vi "Port_set.vi"(8 "error in (no error)":errorcluster, 9 "Port":i32=10002 min=1, 10 "Stream Group":i32=1 min=1, 11 "OXY_SCPI Reseource In":refnum<visa-resource-name>) -> (0 "error out":errorcluster, 1 "communication_data":T1, 3 "OXY_SCPI Reseource Out":refnum<visa-resource-name>)   [LabVIEW 2020, in "OXYGEN_Datastream.lvlib"]
uses:
  OXYGEN_Datastream.lvlib
  TypeDefs/Cluster_RawCommData.ctl
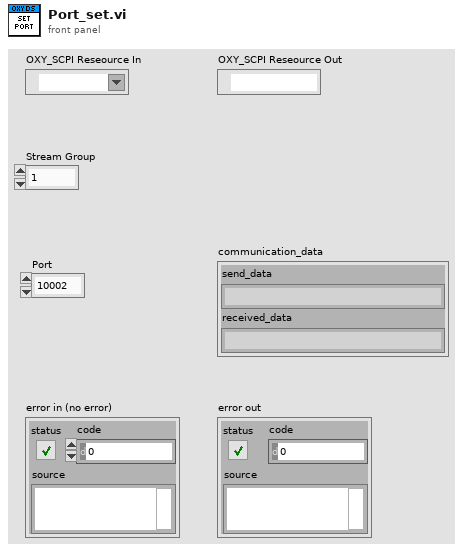
[diagram p1: front panel]
types:
  T1 = typedef "OXYGEN_Datastream.lvlib/Cluster_RawCommData.ctl" = cluster{"send_data":string, "received_data":string}
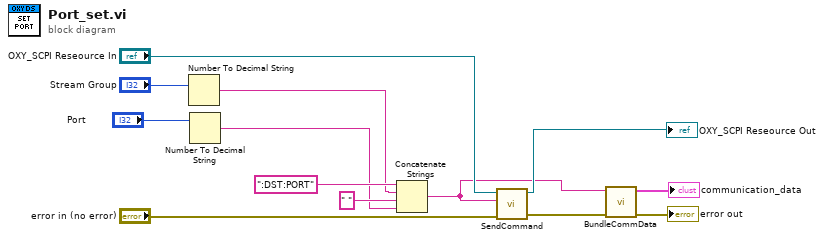
[diagram p0: block diagram]
diagram:
  n1 = Number To Decimal String(number="Stream Group") -> (decimal integer string=w5:string)  [unwired: 1 in]
  n2 = Number To Decimal String(number="Port") -> (decimal integer string=w2:string)  [unwired: 1 in]
  n3 = Concatenate Strings(":DST:PORT", w5, " ", w2) -> (w8:string)
  n4 = call "SendCommand.vi"("error in (no error)"="error in (no error)", "String to Send"=w8, "OXY_SCPI Reseource In"="OXY_SCPI Reseource In") -> ("error out"=w9:errorcluster, "OXY_SCPI Reseource Out"=→"OXY_SCPI Reseource Out":refnum<visa-resource-name>)  [unwired: 7 in]
  n5 = call "BundleCommData.vi"("error in (no error)"=w9, "send_data"=w8) -> ("error out"=→"error out":errorcluster, "communication_data"=→"communication_data":T1)  [unwired: 8 in]
